vi "Set Text.vi"(8 "error in (no error)":errorcluster, 10 "Text":string, 11 "xwpfRun.Figure in":refnum<class "xwpfRun.Figure.lvclass">) -> (0 "error out":errorcluster, 3 "xwpfRun.Figure out":refnum<class "xwpfRun.Figure.lvclass">)   [LabVIEW 2017, in "Word_Specific.lvlib" / "xwpfRun.Figure.lvclass"]
uses:
  xwpfRun.Figure.lvclass
  xwpfRun.Figure.lvclass/xwpfRun.Figure.ctl
  xwpfRun/xwpfRun.lvclass
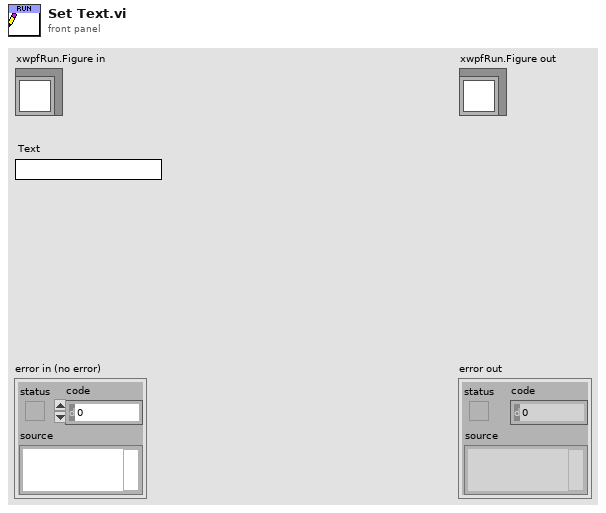
[diagram p1: front panel]
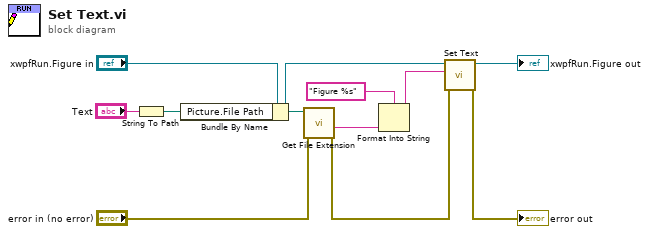
[diagram p0: block diagram]
diagram:
  n1 = String To Path(string="Text") -> (path=w7:path)
  n2 = Bundle By Name(cluster="xwpfRun.Figure in", "Picture.File Path"=w7) -> (w9:refnum<class "xwpfRun.Figure.lvclass">)
  n3 = call <vilib>:"Get File Extension.vi"("error in (no error)"="error in (no error)", "file"=w7) -> ("error out"=w4:errorcluster, "filename without extension"=w3:string)  [unwired: 5 in, 3 out]
  n4 = Format Into String(format string="Figure %s", w3) -> (resulting string=w2:string)  [unwired: 2 in, 1 out]
  n5 = call-parent "Set Text.vi"("error in (no error)"=w4, "Text"=w2, "xwpfRun in"=w9) -> ("error out"=→"error out":errorcluster, "xwpfRun out"=→"xwpfRun.Figure out":refnum<class "xwpfRun.Figure.lvclass">)  [unwired: 7 in]
